vi "Dashboard Main.vi"() -> ()   [LabVIEW 2014]
uses:
  <vilib>/event_ctls.llb/eventvkey.ctl
  <vilib>/Rock Robotics/WPI/Dashboard/WPI_DashboardLogging Global.vi
  <vilib>/Utility/config.llb/Write Key (String).vi
  <vilib>/Utility/config.llb/Write Key (I32).vi
  <vilib>/Rock Robotics/Network Tables/SD Read Boolean.vi
  <vilib>/Rock Robotics/Network Tables/SD Write Number.vi
  <vilib>/Rock Robotics/Network Tables/SD Write Boolean.vi
  <vilib>/Utility/config.llb/NI_LVConfig.lvlib
panel:
  out "VISA resource name out":refnum<visa-resource-name>
  in  "TCP":refnum<k5>
  in  "Rec Mode":enum32{"Stop", "Record", "Playback"}(radio)
  in  "Vision":u16(ring) items=["Camera Off", "USB Camera SW", "USB Camera HW", "IP Camera"]
  out "Image Message":string="Timeout in Camera Communications"
  in  "Dashboard Tab":T1(tab)
  in  "Camera Settings":T2={"Frame Rate"=30, "Compression"=30, "Size"=1} {"Frame Rate" scale=1.0..30.0; "Size" items=["640x480", "320x240", "160x120"]}
  out "MotorChart R":cluster{"Numeric":dbl, "Numeric":dbl}(graph)
  out "MotorChart L":T3(graph)
  out "MotorSliders R":cluster{"MotorSlide1":dbl, "MotorSlide2":dbl} {"MotorSlide2" scale=-1.0..1.0 scale format="%#_2e"; "MotorSlide1" scale=-1.0..1.0 scale format="%#_2e"}
  out "MotorSliders L":T4 {"MotorSlide4 2" scale=0.0..14.0 scale format="%#_2e"; "MotorSlide2" scale=-1.0..1.0 scale format="%#_2e"; "MotorSlide1" scale=-1.0..1.0 scale format="%#_2e"}
  out "Gyro":dbl(knob) scale=0.0..360.0
  out "JS1 Z":dbl(slide) scale=-1.0..1.0 scale format="%#_2e"
  out "JS1 Graph":cluster{"X":dbl, "Y":dbl}[](graph)
  out "JS1 Buttons":T5
  out "JS2 Z":dbl(slide) scale=-1.0..1.0 scale format="%#_2e"
  out "JS2 Graph":cluster{"X":dbl, "Y":dbl}[](graph)
  out "JS2 Buttons":T5
  out "Mode":T6(ring)=enum."Auto Disabled"
  in  "DB Camera Config":bool
  out "fps":dbl format="%#.1g"
  out "Mbps":dbl format="%#.1g"
  out "Mbps 2":bool
  in  "dashButton5":bool
  out "Camera IP":string
  out "Boolean 2":bool
  in  "DB/String 9":string
  in  "DB/String 8":string
  in  "DB/String 7":string
  in  "DB/String 6":string
  in  "DB/String 5":string
  in  "DB/String 4":string
  in  "DB/String 3":string
  in  "DB/String 2":string
  in  "DB/String 1":string
  in  "DB/String 0":string
  in  "DB/Slider 0":dbl(slide) scale=0.0..5.0
  in  "DB/Slider 1":dbl(slide) scale=0.0..5.0
  in  "DB/Slider 2":dbl(slide) scale=0.0..5.0
  in  "DB/Slider 3":dbl(slide) scale=0.0..5.0
  out "DB/LED 3":bool
  out "DB/LED 2":bool
  out "DB/LED 1":bool
  out "DB/LED 0":bool
  in  "DB/Button 3":bool
  in  "DB/Button 2":bool
  in  "DB/Button 1":bool
  in  "DB/Button 0":bool caption="New Name"
  out "error out":errorcluster
  in  "Test Slider":dbl(slide) scale=0.0..100.0 scale format="%#_3g"
  in  "On/Off":bool caption="Solenoid"
  in  "Test Name":u16(ring) items=["Select the test to run...", "Example Test", "-------------------------------", "List of tests is built in robot code.", "Replace with your own automated tests."]
  in  "Test Tree":string(tree)
  in  "Motor":cluster{"Value":dbl, "Enable":bool} {"Value" scale=-1.0..1.0 scale format="%#_3g"}
  out "Progress":T7 {"Test Progress" scale=0.0..100.0}
  in  "Rev/Fwd":cluster{"Forward":bool, "Reverse":bool}
  in  "Test Ring":u16(ring) items=["Monochrome", "Color"]
  in  "Listbox":i32(listbox)
  out "Tree":string(tree)
  out "Camera Image":T8(plugin-control)
  out "Boolean":bool
  # "Left"
  # "Front"
  # "Right"
  # "Battery"
  # "test projectY"
  # "This tab is a great place for autonomous settings and robot-specific values.\nPlace controls and indicators inside this tab and match name to\nDashboard Variables on robot. You can also delete this comment."
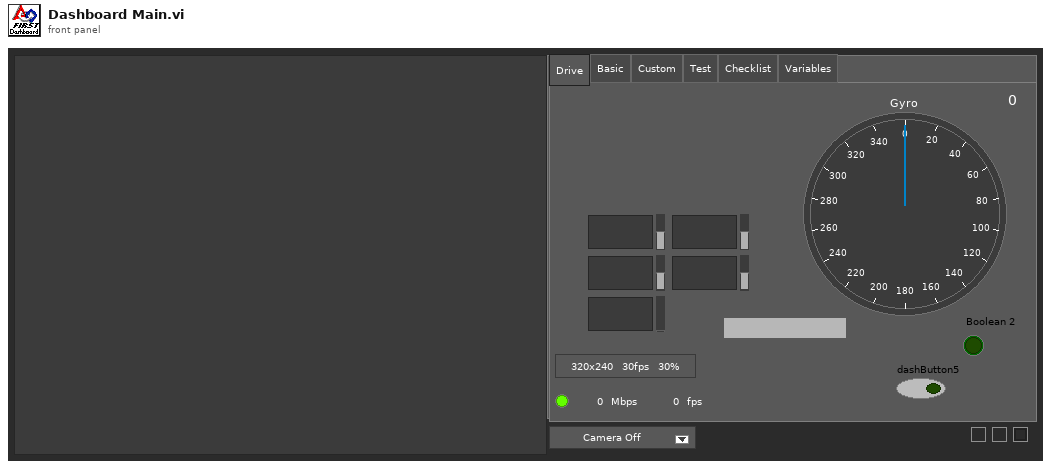
[diagram p1: front panel]
types:
  T1 = enum32{"Drive", "Basic", "Custom", "Test", "Checklist", "Variables"}
  T2 = cluster{"Frame Rate":i32, "Compression":i32, "Size":u16}
  T3 = cluster{"Numeric":dbl, "Numeric":dbl, "Battery V":dbl}
  T4 = cluster{"MotorSlide1":dbl, "MotorSlide2":dbl, "MotorSlide4 2":dbl}
  T5 = cluster{bool, bool, bool, bool, bool, bool, bool, bool, bool, bool, bool, bool}
  T6 = enum8{"Tele-Op Disabled", "Tele-Op Enabled", "Auto Disabled", "Auto Enabled", "Test Disabled", "Test Enabled", "Disconnected", "No Code", "E-Stop"}
  T7 = cluster{"Test Progress":u8, "Test Progress Text":string}
  T8 = typedef "IMAQ Image.ctl" = refnum<image>
  T9 = typedef "Image Type" = u32
  T10 = cluster{"Camera Image":refnum<vi>, "Dashboard Tab":refnum<vi>, "Boolean":refnum<vi>, "Vision":refnum<vi>, "Rec Mode":refnum<vi>, "Test Slider":refnum<vi>, "On/Off ":refnum<vi>, "Test Ring":refnum<vi>, "Rev/Fwd":refnum<vi>, "Test Name":refnum<vi>, "Motor":refnum<vi>, "Progress":refnum<vi>, "CheckList":refnum<vi>, "Tree":refnum<vi>, "Test Tree":refnum<vi>}
  T11 = cluster{"Error Strings":string, "Disable Counts":cluster{u16, u16}, "Rail Faults":cluster{u16, u16, u16}, "Robot IP":string, "DB Mode":u8, "Event Info":cluster{"Name":string, "Type":u8, "Number":u16, "Replay":u8}, "Camera Addr":string}
  T12 = cluster{"Storage":cluster{"Disk Free":u64, "RAM Block":u32, "RAM free":u32}, "CPU Utilization":cluster{"CPU % ISR":sgl, "CPU % Time Crit":sgl, "CPU % Timed Str":sgl, "CPU % High":sgl, "CPU % Above":sgl, "CPU % Normal":sgl, "CPU % Low":sgl}, "CAN":cluster{"% Bus Utilization":sgl, "Bus Off Cnt":u32, "TX_FIFO Full Cnt":u32, "Receive Error Cnt":u8, "Transmit Error Cnt":u8}, "HID":cluster{"HID Outputs":u32, "Rumble Low":u16, "Rumble High":u16}[]}
  T13 = cluster{"Status bits":cluster{"Test Mode":bool, "Autonomous":bool, "Enabled":bool, "Code Start":bool, "Brownout":bool, "Reserved 2":bool, "Reserved 3":bool, "E-Stop":bool}, "Code Trace":cluster{"Disabled":bool, "TeleOp":bool, "Auto":bool, "Test":bool}, "Controller Type":enum16{"unknown", "cRIO", "roboRio"}, "Code?":enum16{"unknown", "noCode", "code"}, "Battery V":dbl}
  T14 = cluster{"Control Bits":cluster{"TestMode":bool, "Autonomous":bool, "Enabled":bool, "FMS Present":bool, bool, bool, bool, "E-Stop":bool}, "Team Station ":u8, "Countdown":sgl, "Joystick Values":cluster{"Axes":dbl[], "Buttons":bool[], "POVs":i16[]}[]}
  T15 = cluster{"Axes":dbl[], "Buttons":bool[], "POVs":i16[]}[]
  T16 = cluster{"Axes":dbl[], "Buttons":bool[], "POVs":i16[]}
  T17 = cluster{"Buttons[0]":bool, "Buttons[1]":bool, "Buttons[2]":bool, "Buttons[3]":bool, "Buttons[4]":bool, "Buttons[5]":bool, "Buttons[6]":bool, "Buttons[7]":bool, "Buttons[8]":bool, "Buttons[9]":bool, "Buttons[10]":bool, "Buttons[11]":bool}
  T18 = cluster{"pickup":dbl, "1tote":dbl, "2tote":dbl, "3tote":dbl, "1container":dbl, "1container1tote":dbl, "1container2tote":dbl, "1container3tote":dbl}
  T19 = typedef "NI_LVConfig.lvlib/Config Data RefNum.ctl" = refnum<k1>
  T20 = cluster{"Operation":enum16{"Update", "Clear"}, "Color Box":u32}[]
  T21 = typedef "eventvkey.ctl" = enum16{"ASCII", "Enter", "Return", "Shift", "Ctrl", "Alt", "Cmd", "Opt", "Caps", "NumLock", "Clear", "Break", "Up", "Down", "Left", "Right", "Insert", "Delete", "Home", "End", "PageUp", "PageDown", "Escape", "Help", "Pause", "ScrollLock", "F1", "F2", "F3", "F4", "F5", "F6", "F7", "F8", "F9", "F10", "F11", "F12", "F13", "F14", "F15", "F16", "F17", "F18", "F19", "F20", "F21", "F22", "F23", "F24", "Play", "VolumeUp", "VolumeDown", "Mute", "Two Byte Char"}
  T22 = cluster{"Image Size":bool, "Image Type":bool, "Pixel Value":bool, "ROI Information":bool, "Zoom Factor":bool}
  T23 = enum8{"Enabled", "Disabled", "Disabled and Grayed Out"}
  T24 = cluster{"Operation":enum16{"Update", "Clear"}, "Color Box":u32}
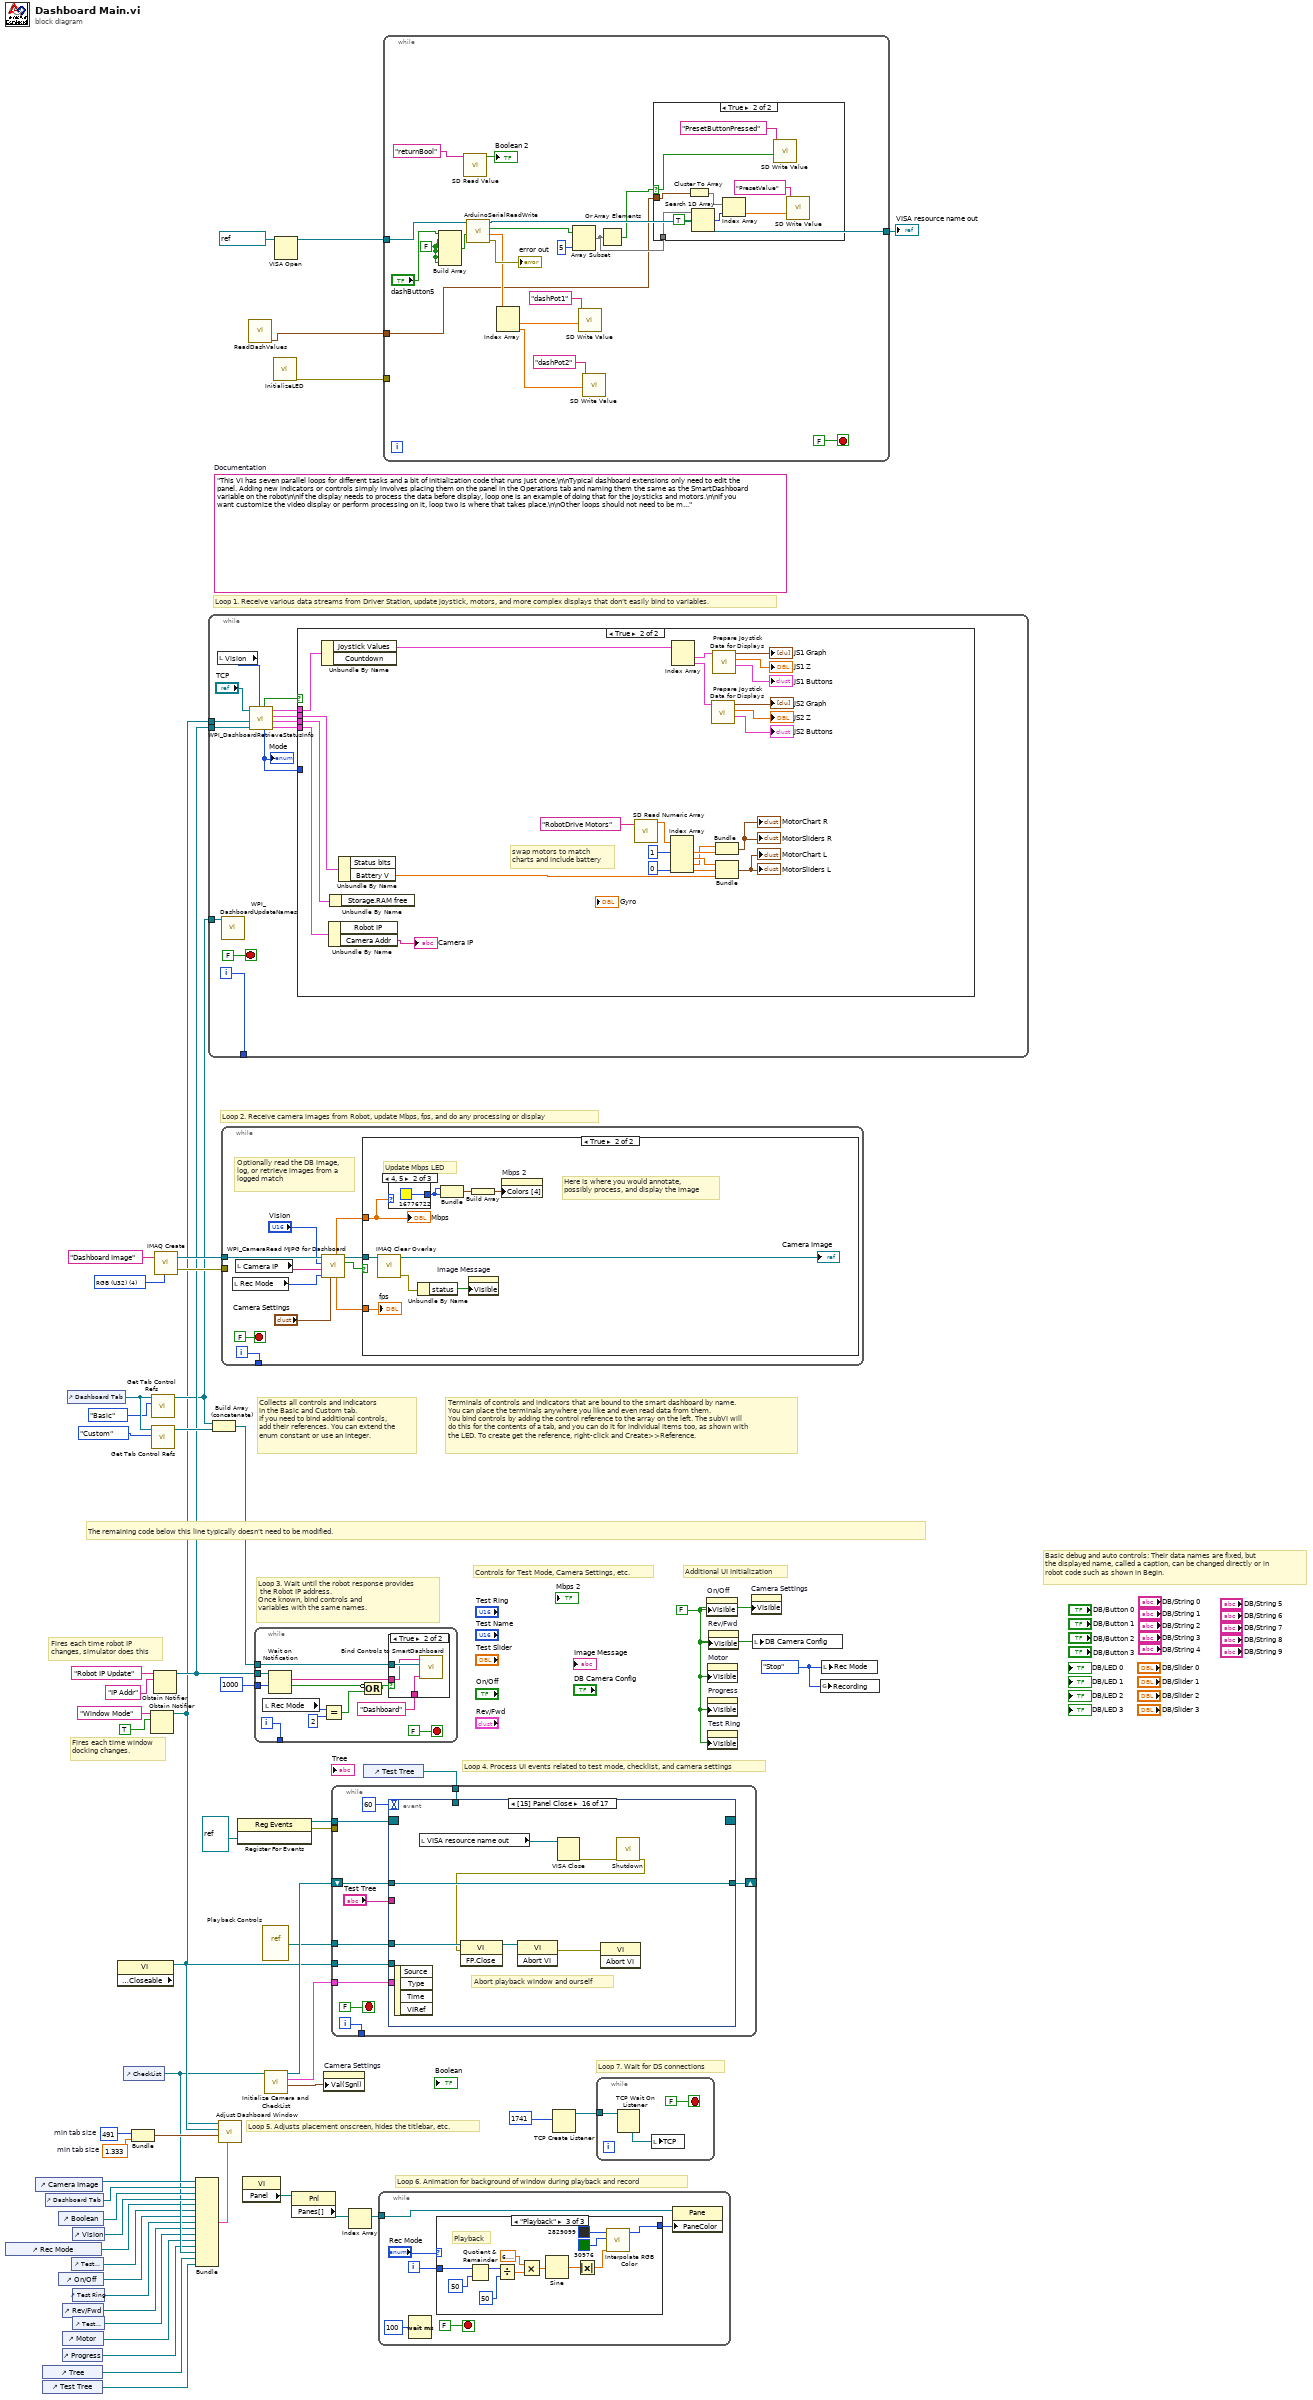
[diagram p0: block diagram]
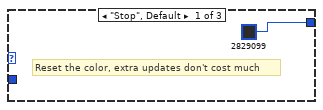
[diagram p4: hidden frame]
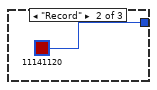
[diagram p5: hidden frame]
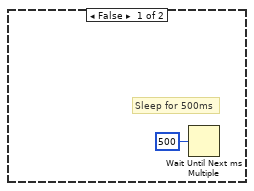
[diagram p7: hidden frame]
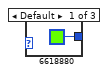
[diagram p8: hidden frame]
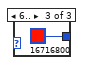
[diagram p9: hidden frame]
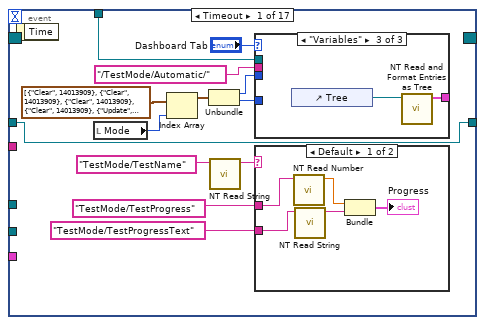
[diagram p10: hidden frame]
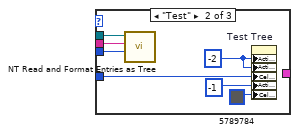
[diagram p12: hidden frame]
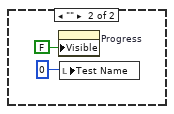
[diagram p13: hidden frame]
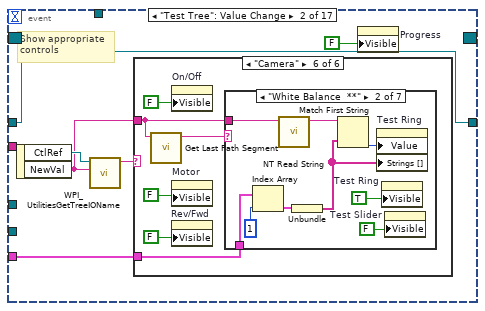
[diagram p14: hidden frame]
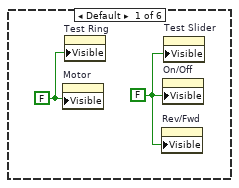
[diagram p15: hidden frame]
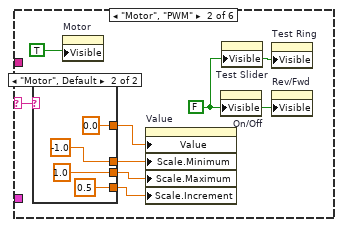
[diagram p16: hidden frame]
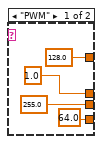
[diagram p17: hidden frame]
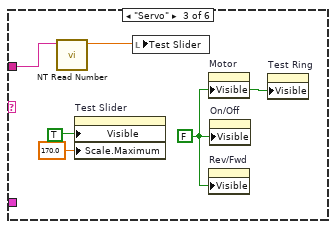
[diagram p18: hidden frame]
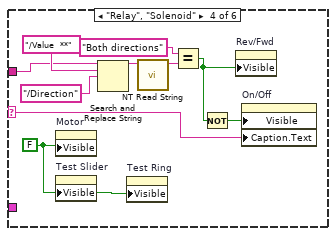
[diagram p19: hidden frame]
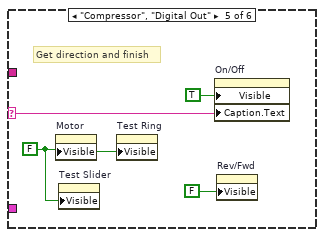
[diagram p20: hidden frame]
diagram:
  w29 = 491  # min tab size
  w28 = 1.333  # min tab size
  w37 = enum32{"Stop", "Record", "Playback"}."Stop" ("Rec Mode")
  w11 = FALSE ("Visible")
  (unwired) "This VI has seven parallel loops for different tasks and a bit of initialization code that runs just once.\n\nTypical dashboard extensions only need to edit the panel. Adding new indicators or controls simply involves placing them on the panel in the Operations tab and naming them the same as the SmartDashboard variable on the robot\n\nIf the display needs to process the data before display, loop one is an example of doing that for the joysticks and motors.\n\nIf you want customize the video display or perform processing on it, loop two is where that takes place.\n\nOther loops should not need to be modified. They are pretty standard, and document the task they perform."  # Documentation
  w57 = T9 4 items=["Grayscale (U8)", "Grayscale (I16)", "Grayscale (SGL)", "Complex (CSG)", "RGB (U32)", "HSL (U32)", "RGB (U64)"] ("Image Type")
  # "Loop 7. Wait for DS connections"
  # "Basic debug and auto controls: Their data names are fixed, but\nthe displayed name, called a caption, can be changed directly or in\nrobot code such as shown in Begin."
  # "Controls for Test Mode, Camera Settings, etc."
  # "Additional UI Initialization"
  # "Loop 6. Animation for background of window during playback and record"
  # "Fires each time robot IP\nchanges, simulator does this"
  # "Fires each time window\ndocking changes."
  # "Collects all controls and indicators\nin the Basic and Custom tab.\nIf you need to bind additional controls,\nadd their references. You can extend the\nenum constant or use an integer."
  # "The remaining code below this line typically doesn't need to be modified."
  # "Loop 4. Process UI events related to test mode, checklist, and camera settings"
  # "Terminals of controls and indicators that are bound to the smart dashboard by name.\nYou can place the terminals anywhere you like and even read data from them.\nYou bind controls by adding the control reference to the array on the left. The subVI will\ndo this for the contents of a tab, and you can do it for individual items too, as shown with\nthe LED. To create get the reference, right-click and Create>>Reference."
  # "Loop 3. Wait until the robot response provides\n the Robot IP address.\nOnce known, bind controls and\nvariables with the same names."
  # "Loop 5. Adjusts placement onscreen, hides the titlebar, etc."
  # "Loop 1. Receive various data streams from Driver Station, update joystick, motors, and more complex displays that don't easily bind to variables."
  # "Loop 2. Receive camera images from Robot, update Mbps, fps, and do any processing or display"
  n1 = control-ref of="Rec Mode"() -> (w17:refnum<vi>)
  n2 = control-ref of="Camera Image"() -> (w32:refnum<vi>)
  n3 = control-ref of="Tree"() -> (w21:refnum<vi>)
  n4 = control-ref of="Test Tree"() -> (w20:refnum<vi>)
  n5 = control-ref of="Dashboard Tab"() -> (w31:refnum<vi>)
  n6 = control-ref of="Boolean"() -> (w26:refnum<vi>)
  n7 = control-ref of="On/Off"() -> (w15:refnum<vi>)
  n8 = control-ref of="Progress"() -> (w12:refnum<vi>)
  n9 = control-ref of="Rev/Fwd"() -> (w13:refnum<vi>)
  n10 = control-ref of="Motor"() -> (w18:refnum<vi>)
  n11 = control-ref of="Dashboard Tab"() -> (w35:refnum<vi>)
  n12 = control-ref of="Test Slider"() -> (w16:refnum<vi>)
  n13 = control-ref of="Vision"() -> (w30:refnum<vi>)
  n14 = control-ref of="Test Ring"() -> (w14:refnum<vi>)
  n15 = control-ref of="Test Name"() -> (w19:refnum<vi>)
  n16 = property class="VI" props=["Front Panel.Closeable"]() -> (reference out=w36:refnum<vi>)  [unwired: 2 in, 2 out]
  n17 = control-ref of="CheckList"() -> (w22:refnum<vi>)
  n18 = Bundle("min tab size"=w29, "min tab size"=w28) -> (w27:cluster{"min tab size":i32, "min tab size":dbl})  [unwired: 1 in]
  n19 = Obtain Notifier(name (unnamed)="Window Mode", notification data type=TRUE) -> (notifier out=w8:refnum<notifier>)  [unwired: 2 in, 2 out]
  n20 = call <vilib>:"Get Tab Control Refs.vi"("Page Index"=T1."Basic" ("Dashboard Tab"), "TabControl in"=w35) -> ("ControlsOnPage"=w9:refnum<vi>[])  [unwired: 9 in]
  n21 = call <vilib>:"Get Tab Control Refs.vi"("Page Index"=T1."Custom" ("Dashboard Tab"), "TabControl in"=w35) -> ("ControlsOnPage"=w34:refnum<vi>[])  [unwired: 9 in]
  n22 = Obtain Notifier(name (unnamed)="Robot IP Update", notification data type="IP Addr" ("name (unnamed)")) -> (notifier out=w10:refnum<notifier>)  [unwired: 2 in, 2 out]
  n23 = call "IMAQ Create"("Image Name"="Dashboard Image", "Image Type"=w57) -> ("New Image"=w55:T8, "error out"=w54:errorcluster)  [unwired: 2 in, 1 out]
  n24 = Bundle("Camera Image"=w32, "Dashboard Tab"=w31, "Boolean"=w26, "Vision"=w30, "Rec Mode"=w17, "Test Slider"=w16, "On/Off"=w15, "Test Ring"=w14, "Rev/Fwd"=w13, "Test Name"=w19, "Motor"=w18, "Progress"=w12, "CheckList"=w22, "Tree"=w21, "Test Tree"=w20) -> (w23:T10)  [unwired: 1 in]
  n25 = while {
    tunnel: [w69] -> _
    tunnel: w10 -> [w63]
    tunnel: w9 -> [w62]
    tunnel: w8 -> [w58]
    i -> [w69]
    stop <- FALSE stop-if-true
    n26 = local read "Vision"() -> (w60:u16)
    n27 = call <vilib>:"WPI_DashboardUpdateNames.vi"("Controls on Tab"=w62) -> ()  [unwired: 11 in]
    n28 = call <vilib>:"WPI_DashboardRetrieveStatusInfo.vi"("Vision"=w60, "Binding Refnum"=w63, "Window Mode Notifier"=w58, "TCP Cnx"="TCP") -> ("Power and Errors"=w64:T11, "Robot Metrics"=w67:T12, "Status Info"=w68:T13, "Control Info"=w65:T14, "Robot Mode"=w61:T6, "Process?"=w66:bool)  [unwired: 2 in]
    "Mode" <- w61
    n29 = case shown="True" w66 {
      tunnel: w68 -> [_ w95]
      tunnel: w67 -> [_ w94]
      tunnel: w65 -> [_ w93]
      tunnel: w64 -> [_ w92]
      tunnel: w61 -> [_ _]
      frame False {
      }
      frame True {
        # "swap motors to match\ncharts and include battery"
        n30 = Unbundle By Name(w93) -> ("Joystick Values"=w80:T15)  [unwired: 1 out]
        n31 = Unbundle By Name(w92) -> ("Camera Addr"=→"Camera IP":string)  [unwired: 1 out]
        n32 = Unbundle By Name(w94) -> ()  [unwired: 1 out]
        n33 = Unbundle By Name(w95) -> ("Battery V"=w81:dbl)  [unwired: 1 out]
        n34 = call <vilib>:"SD Read Numeric Array.vi"("Name"="RobotDrive Motors") -> ("Numeric Array"=w83:dbl[])  [unwired: 8 in, 2 out]
        n35 = Index Array(array=w83, index #1=1, index #4=0) -> (element #1=w87:dbl, element #2=w88:dbl, element #3=w86:dbl, element #4=w91:dbl)  [unwired: 2 in]
        n36 = Index Array(array=w80) -> (element #1=w79:T16, element #2=w74:T16)  [unwired: 2 in]
        n37 = call "Prepare Joystick Data for Displays.vi"("Joystick Values"=w74) -> ("Buttons"=→"JS2 Buttons":T17, "Z Axis"=→"JS2 Z":dbl, "Cartesian Data"=→"JS2 Graph":cluster{"X axis":dbl, "X axis":dbl}[])  [unwired: 8 in]
        n38 = call "Prepare Joystick Data for Displays.vi"("Joystick Values"=w79) -> ("Buttons"=→"JS1 Buttons":T17, "Z Axis"=→"JS1 Z":dbl, "Cartesian Data"=→"JS1 Graph":cluster{"X axis":dbl, "X axis":dbl}[])  [unwired: 8 in]
        n39 = Bundle("Numeric"=w86, "Numeric"=w87) -> (→"MotorChart R" →"MotorSliders R":cluster{"Numeric":dbl, "Numeric":dbl})  [unwired: 1 in]
        n40 = Bundle("Numeric"=w88, "Numeric"=w91, "Battery V"=w81) -> (→"MotorChart L" →"MotorSliders L":T3)  [unwired: 1 in]
      }
    }
  }
  n41 = Build Array (concatenate)(w9, w34) -> (w33:refnum<vi>[])
  n42 = call "Adjust Dashboard Window.vi"("Sizing Refnums"=w23, "Size Constraints"=w27, "VI"=w36, "Notifier in"=w8) -> ()  [unwired: 8 in]
  n43 = while {
    tunnel: w55 -> [w104]
    tunnel: w54 -> [_]
    tunnel: [w105] -> _
    i -> [w105]
    stop <- FALSE stop-if-true
    # "Optionally read the DB image,\nlog, or retrieve images from a\nlogged match"
    n44 = local read "Rec Mode"() -> (w98:enum32{"Stop", "Record", "Playback"})
    n45 = local read "Camera IP"() -> (w96:string)
    n46 = call <vilib>:"WPI_CameraRead MJPG for Dashboard.vi"("Camera Settings"="Camera Settings", "Rec Mode"=w98, "Camera IP"=w96, "Camera Mode"="Vision", "Refnum in"=w104) -> ("Active"=w102:bool, "Refnum out"=w103:T8, "FPS"=w101:dbl, "Bandwidth (Mbps)"=w100:dbl)  [unwired: 3 in]
    n47 = case shown="True" w102 {
      tunnel: w103 -> [_ w111]
      tunnel: w100 -> [_ w110]
      tunnel: w101 -> [_ w108]
      frame False {
        # "Sleep for 500ms"
        n48 = Wait Until Next ms Multiple(millisecond multiple=u32 500) -> ()  [unwired: 1 out]
      }
      frame True {
        # "Here is where you would annotate,\npossibly process, and display the image"
        # "Update Mbps LED"
        n49 = call "IMAQ Clear Overlay"("Image"=w111) -> ("error out"=w115:errorcluster, "Image Out"=→"Camera Image":T8)  [unwired: 2 in, 7 out]
        n50 = case shown="4, 5" w110 {
          tunnel: [u32 6618880 ("Color Box") u32 16776722 ("Color Box") u32 16716800 ("Color Box")] -> w112
          frame Default {
          }
          frame 4, 5 {
          }
          frame 6.. {
          }
        }
        n51 = Unbundle By Name(w115) -> ("status"=w116:bool)
        n52 = Bundle("Color Box"=w112, "Color Box"=w112) -> (w114:cluster{"Color Box":u32, "Color Box":u32})  [unwired: 1 out]
        n53 = property on="Image Message" class="Str"("Visible"=w116) -> ()  [unwired: 2 in, 2 out]
        n54 = Build Array(w114) -> (w113:cluster{"Color Box":u32, "Color Box":u32}[])
        n55 = property on="Mbps 2" class="Bool (strict)"("Colors [4]"=w113) -> ()  [unwired: 2 in, 2 out]
        "Mbps" <- w110
        "fps" <- w108
      }
    }
  }
  n56 = register-events(refnum<vi> refnum) -> (reference out=w41:refnum<event-registration>, error out=w40:errorcluster)  [unwired: 2 in]
  n57 = property class="VI"() -> ("Panel"=w44:refnum<vi>)  [unwired: 2 in, 2 out]
  n58 = call "ReadDashValues.vi"() -> ("output cluster"=w2:T18)  [unwired: 11 in]
  n59 = while {
    tunnel: w33 -> [w131]
    tunnel: w10 -> [w129]
    tunnel: [w127] -> _
    tunnel: u32 1000 ("milliseconds to wait") -> [w126]
    i -> [w127]
    stop <- FALSE stop-if-true
    n60 = local read "Rec Mode"() -> (w122:enum32{"Stop", "Record", "Playback"})
    n61 = Wait on Notification(notifier=w129, timeout in ms (-1)=w126) -> (notification=w128:string, timed out?=w124:bool)  [unwired: 2 in, 2 out]
    n62 = Equal?(x=w122, y=u16 2 ("Rec Mode")) -> (x = y?=w123:bool)
    n63 = Compound Arithmetic op=OR(invert w124, w123) -> (w125:bool)
    n64 = case shown="True" w125 {
      tunnel: w131 -> [_ w134]
      tunnel: w128 -> [_ w133]
      tunnel: "Dashboard" -> [_ w132]
      frame False {
      }
      frame True {
        n65 = call <vilib>:"Bind Controls to SmartDashboard.vi"("Client Name"=w132, "Bound Control Refs"=w134, "Server IP Address"=w133) -> ()  [unwired: 9 in]
      }
    }
  }
  n66 = vi-ref "Playback Controls.vi"() -> (w42:refnum<vi>)
  n67 = call "Initialize Camera and CheckList.vi"("ListBox in"=w22) -> ("Cluster"=w48:cluster{"value":i32, "value":i32, "index":i32}, "Array"=w49:cluster{string[]}[], "File Refnum"=w47:T19)  [unwired: 8 in]
  n68 = call "InitializeLED.vi"() -> ("error out"=w1:errorcluster)  [unwired: 11 in]
  n69 = VISA Open(VISA resource name=refnum<visa-resource-name> "COM3") -> (VISA resource name=w4:refnum<visa-resource-name>)  [unwired: 4 in, 1 out]
  n70 = property class="Pnl"(reference=w44) -> ("Panes[]"=w45:refnum<vi>[])  [unwired: 1 in, 2 out]
  n71 = property on="Camera Settings" class="Clust (strict)"("Val(Sgnl)"=w48) -> ()  [unwired: 2 in, 2 out]
  n72 = Index Array(array=w45) -> (element=w43:refnum<vi>)  [unwired: 1 in]
  n73 = control-ref of="Test Tree"() -> (w46:refnum<vi>)
  n74 = while {
    tunnel: w49 -> [w142]
    shift-right: [w141] -> _
    shift-left: w47 -> [w140]
    tunnel: [w139] -> _
    tunnel: w46 -> [w138]
    tunnel: w42 -> [w137]
    tunnel: w41 -> [w136]
    tunnel: w40 -> [_]
    tunnel: w36 -> [w135]
    i -> [w139]
    stop <- FALSE stop-if-true
    n75 = event shown="[15] Panel Close" {
      selector: w136 -> [_ _ _ _ _ _ _ _ _ _ _ _ _ _ _ _ _]
      dyn-events: [_ _ _ _ _ _ _ _ _ _ _ _ _ w380 _ _ _] -> _
      timeout: u32 60 ("milliseconds to wait") -> [_ _ _ _ _ _ _ _ _ _ _ _ _ _ _ _ _]
      tunnel: w138 -> [w154 _ _ _ _ _ _ _ _ _ _ _ _ _ _ _ _]
      tunnel: "Test Tree" -> [_ _ _ _ _ _ _ _ w349 w357 w359 w363 w371 _ _ _ _]
      tunnel: w142 -> [_ w176 _ _ _ _ w313 w343 _ _ _ _ _ _ _ _ _]
      tunnel: [w150 w175 w274 w279 w287 w299 w312 w336 w348 w355 w358 w362 w370 w382 w396 w400 w410] -> w141
      tunnel: w140 -> [w150 w175 w274 w279 w287 w299 w311 w336 w348 w355 w358 w362 w370 w382 w396 w400 w410]
      tunnel: w137 -> [_ _ _ _ _ _ _ _ _ _ _ _ _ w383 _ w403 _]
      tunnel: w135 -> [_ _ _ _ _ _ _ _ _ _ _ _ _ w378 _ _ _]
      event Timeout {
        n76 = event-data() -> ()  [unwired: 1 in, 1 out]
        n77 = local read "Mode"() -> (w153:T6)
        n78 = Index Array(array=T20 [{"Operation"=enum."Clear", "Color Box"=14013909}, {"Operation"=enum."Clear", "Color Box"=14013909}, {"Operation"=enum."Clear", "Color Box"=14013909}, {"Operation"=enum."Clear", "Color Box"=14013909}, {"Operation"=enum."Update", "Color Box"=14013909}, {"Operation"=enum."Update", "Color Box"=16777215}, {"Operation"=enum."Clear", "Color Box"=14013909}, {"Operation"=enum."Clear", "Color Box"=14013909}, {"Operation"=enum."Clear", "Color Box"=14013909}], index=w153) -> (element=w148:T24)
        n79 = Unbundle(w148) -> ("Operation"=w147:enum16{"Update", "Clear"}, "Color Box"=w146:u32)
        n80 = call <vilib>:"NT Read String.vi"("Name"="TestMode/TestName") -> ("String"=w157:string)  [unwired: 9 in, 1 out]
        n81 = case shown="\"Variables\"" "Dashboard Tab" {
          tunnel: w154 -> [_ w165 _]
          tunnel: "/TestMode/Automatic/" ("Name Pattern") -> [_ w164 _]
          tunnel: w147 -> [_ w163 _]
          tunnel: [_ _ w167] -> _
          tunnel: w146 -> [_ w159 _]
          frame "Custom", Default {
          }
          frame "Test" {
            w162 = -2 ("Active Item:Row Number")
            n82 = call <vilib>:"NT Read and Format Entries as Tree.vi"("Operation"=w163, "Name Pattern"=w164, "Tree Refnum"=w165) -> ()  [unwired: 7 in, 2 out]
            n83 = property on="Test Tree" class="Tree (strict)"("Active Item Row Number"=w162, "ActiveColNum"=w162, "CellBG"=w159, "Active Item Row Number"=-1 ("Active Item:Row Number"), "CellBG"=u32 5789784 ("Color Box")) -> ()  [unwired: 2 in, 2 out]
          }
          frame "Variables" {
            n84 = control-ref of="Tree"() -> (w166:refnum<vi>)
            n85 = call <vilib>:"NT Read and Format Entries as Tree.vi"("Tree Refnum"=w166) -> ("Formatted Strings"=w167:cluster{"Name":string, "Value":string}[])  [unwired: 9 in, 1 out]
          }
        }
        n86 = case shown="Default" w157 {
          tunnel: "TestMode/TestProgress" ("Name") -> [w169 _]
          tunnel: "TestMode/TestProgressText" ("Name") -> [w168 _]
          frame Default {
            n87 = call <vilib>:"NT Read Number.vi"("Name"=w169) -> ("Numeric"=w170:dbl)  [unwired: 9 in, 1 out]
            n88 = call <vilib>:"NT Read String.vi"("Name"=w168) -> ("String"=w171:string)  [unwired: 9 in, 1 out]
            n89 = Bundle("Numeric"=w170, "String"=w171) -> (→"Progress":cluster{"Numeric":dbl, "String":string})  [unwired: 1 in]
          }
          frame "" {
            n90 = property on="Progress" class="Clust (strict)"("Visible"=FALSE) -> ()  [unwired: 2 in, 2 out]
            n91 = local write "Test Name"(u16 0) -> ()
          }
        }
      }
      event "Test Tree": Value Change {
        # "Show appropriate\ncontrols"
        n92 = event-data() -> ("CtlRef"=w179:refnum<vi>, "NewVal"=w177:string)  [unwired: 1 in]
        n93 = call <vilib>:"WPI_UtilitiesGetTreeIOName.vi"("NewVal"=w177, "TreeControl in"=w179) -> ("I/O Name"=w180:string)  [unwired: 9 in]
        n94 = case shown="\"Camera\"" w180 {
          selector: w180 -> [_ w187 _ w205 w214 _]
          tunnel: w177 -> [_ _ w202 w204 _ w221]
          tunnel: w176 -> [_ _ _ _ _ w220]
          frame Default {
            w182 = FALSE ("Visible")
            w181 = FALSE ("Visible")
            n95 = property on="Motor" class="Clust (strict)"("Visible"=w181) -> ()  [unwired: 2 in, 2 out]
            n96 = property on="Test Ring" class="Ring (strict)"("Visible"=w181) -> ()  [unwired: 2 in, 2 out]
            n97 = property on="Rev/Fwd" class="Clust (strict)"("Visible"=w182) -> ()  [unwired: 2 in, 2 out]
            n98 = property on="On/Off" class="Bool (strict)"("Visible"=w182) -> ()  [unwired: 2 in, 2 out]
            n99 = property on="Test Slider" class="Slide (strict)"("Visible"=w182) -> ()  [unwired: 2 in, 2 out]
          }
          frame "Motor", "PWM" {
            w188 = FALSE ("Visible")
            n100 = case shown="\"Motor\", Default" w187 {
              tunnel: [1.0 ("Value") -1.0 ("Value")] -> w186
              tunnel: [255.0 ("Value") 1.0 ("Value")] -> w185
              tunnel: [128.0 ("Value") 0.0 ("Value")] -> w184
              tunnel: [64.0 ("Value") 0.5 ("Value")] -> w183
              frame "PWM" {
              }
              frame "Motor", Default {
              }
            }
            n101 = property on="Motor" class="Clust (strict)"("Visible"=TRUE) -> ()  [unwired: 2 in, 2 out]
            n102 = property on="Value" class="Slide (strict)"("Value"=w184, "Scale.Minimum"=w186, "Scale.Maximum"=w185, "Scale.Increment"=w183) -> ()  [unwired: 2 in, 2 out]
            n103 = property on="On/Off" class="Bool (strict)"("Visible"=w188) -> ()  [unwired: 2 in, 2 out]
            n104 = property on="Test Slider" class="Slide (strict)"("Visible"=w188) -> ()  [unwired: 2 in, 2 out]
            n105 = property on="Test Ring" class="Ring (strict)"("Visible"=w188) -> ()  [unwired: 2 in, 2 out]
            n106 = property on="Rev/Fwd" class="Clust (strict)"("Visible"=w188) -> ()  [unwired: 2 in, 2 out]
          }
          frame "Servo" {
            w200 = FALSE ("Visible")
            n107 = call <vilib>:"NT Read Number.vi"("Name"=w202) -> ("Numeric"=w201:dbl)  [unwired: 9 in, 1 out]
            n108 = property on="Test Slider" class="Slide (strict)"("Visible"=TRUE, "Scale.Maximum"=170.0 ("Scale.Range:Maximum")) -> ()  [unwired: 2 in, 2 out]
            n109 = local write "Test Slider"(w201) -> ()
            n110 = property on="Motor" class="Clust (strict)"("Visible"=w200) -> ()  [unwired: 2 in, 2 out]
            n111 = property on="Rev/Fwd" class="Clust (strict)"("Visible"=w200) -> ()  [unwired: 2 in, 2 out]
            n112 = property on="On/Off" class="Bool (strict)"("Visible"=w200) -> ()  [unwired: 2 in, 2 out]
            n113 = property on="Test Ring" class="Ring (strict)"("Visible"=w200) -> ()  [unwired: 2 in, 2 out]
          }
          frame "Relay", "Solenoid" {
            w203 = FALSE ("Visible")
            n114 = property on="Motor" class="Clust (strict)"("Visible"=w203) -> ()  [unwired: 2 in, 2 out]
            n115 = property on="Test Slider" class="Slide (strict)"("Visible"=w203) -> ()  [unwired: 2 in, 2 out]
            n116 = Search and Replace String(input string=w204, search string="/Value  **", replace string="/Direction") -> (result string=w210:string)  [unwired: 5 in, 3 out]
            n117 = property on="Test Ring" class="Ring (strict)"("Visible"=w203) -> ()  [unwired: 2 in, 2 out]
            n118 = call <vilib>:"NT Read String.vi"("Name"=w210) -> ("String"=w208:string)  [unwired: 9 in, 1 out]
            n119 = Equal?(x="Both directions", y=w208) -> (x = y?=w206:bool)
            n120 = Not(x=w206) -> (.not. x?=w207:bool)
            n121 = property on="Rev/Fwd" class="Clust (strict)"("Visible"=w206) -> ()  [unwired: 2 in, 2 out]
            n122 = property on="On/Off" class="Bool (strict)"("Visible"=w207, "Caption.Text"=w205) -> ()  [unwired: 2 in, 2 out]
          }
          frame "Compressor", "Digital Out" {
            w213 = FALSE ("Visible")
            # "Get direction and finish"
            n123 = property on="Motor" class="Clust (strict)"("Visible"=w213) -> ()  [unwired: 2 in, 2 out]
            n124 = property on="Test Slider" class="Slide (strict)"("Visible"=w213) -> ()  [unwired: 2 in, 2 out]
            n125 = property on="Test Ring" class="Ring (strict)"("Visible"=w213) -> ()  [unwired: 2 in, 2 out]
            n126 = property on="On/Off" class="Bool (strict)"("Visible"=TRUE, "Caption.Text"=w214) -> ()  [unwired: 2 in, 2 out]
            n127 = property on="Rev/Fwd" class="Clust (strict)"("Visible"=FALSE) -> ()  [unwired: 2 in, 2 out]
          }
          frame "Camera" {
            n128 = call <vilib>:"Get Last Path Segment.vi"("String in"=w221) -> ("String out"=w222:string)  [unwired: 10 in]
            n129 = property on="On/Off" class="Bool (strict)"("Visible"=FALSE) -> ()  [unwired: 2 in, 2 out]
            n130 = property on="Motor" class="Clust (strict)"("Visible"=FALSE) -> ()  [unwired: 2 in, 2 out]
            n131 = property on="Rev/Fwd" class="Clust (strict)"("Visible"=FALSE) -> ()  [unwired: 2 in, 2 out]
            n132 = case shown="\"White Balance  **\"" w222 {
              tunnel: w221 -> [w228 w237 w246 w255 w264 _ w270]
              tunnel: w220 -> [w226 w234 w243 w252 w261 _ _]
              frame "Size  **" {
                n133 = Index Array(array=w226) -> (element=w225:cluster{string[]})  [unwired: 1 in]
                n134 = call <vilib>:"NT Read String.vi"("Name"=w228) -> ("String"=w227:string)  [unwired: 9 in, 1 out]
                n135 = Unbundle(w225) -> (w223:string[])
                n136 = Match First String(2:w223, 3:w227) -> (0:w224:i32)  [unwired: 1 out]
                n137 = property on="Test Ring" class="Ring (strict)"("Value"=w224, "Strings []"=w223) -> ()  [unwired: 2 in, 2 out]
                n138 = property on="Test Ring" class="Ring (strict)"("Visible"=TRUE) -> ()  [unwired: 2 in, 2 out]
                n139 = property on="Test Slider" class="Slide (strict)"("Visible"=FALSE) -> ()  [unwired: 2 in, 2 out]
              }
              frame "White Balance  **" {
                n140 = Index Array(array=w234, index=1) -> (element=w235:cluster{string[]})
                n141 = call <vilib>:"NT Read String.vi"("Name"=w237) -> ("String"=w236:string)  [unwired: 9 in, 1 out]
                n142 = Unbundle(w235) -> (w232:string[])
                n143 = Match First String(2:w232, 3:w236) -> (0:w231:i32)  [unwired: 1 out]
                n144 = property on="Test Ring" class="Ring (strict)"("Value"=w231, "Strings []"=w232) -> ()  [unwired: 2 in, 2 out]
                n145 = property on="Test Ring" class="Ring (strict)"("Visible"=TRUE) -> ()  [unwired: 2 in, 2 out]
                n146 = property on="Test Slider" class="Slide (strict)"("Visible"=FALSE) -> ()  [unwired: 2 in, 2 out]
              }
              frame "Exposure  **" {
                n147 = Index Array(array=w243, index=2) -> (element=w244:cluster{string[]})
                n148 = call <vilib>:"NT Read String.vi"("Name"=w246) -> ("String"=w245:string)  [unwired: 9 in, 1 out]
                n149 = Unbundle(w244) -> (w240:string[])
                n150 = Match First String(2:w240, 3:w245) -> (0:w241:i32)  [unwired: 1 out]
                n151 = property on="Test Ring" class="Ring (strict)"("Value"=w241, "Strings []"=w240) -> ()  [unwired: 2 in, 2 out]
                n152 = property on="Test Ring" class="Ring (strict)"("Visible"=TRUE) -> ()  [unwired: 2 in, 2 out]
                n153 = property on="Test Slider" class="Slide (strict)"("Visible"=FALSE) -> ()  [unwired: 2 in, 2 out]
              }
              frame "Exposure Priority  **" {
                n154 = Index Array(array=w252, index=3) -> (element=w253:cluster{string[]})
                n155 = call <vilib>:"NT Read String.vi"("Name"=w255) -> ("String"=w254:string)  [unwired: 9 in, 1 out]
                n156 = Unbundle(w253) -> (w249:string[])
                n157 = Match First String(2:w249, 3:w254) -> (0:w250:i32)  [unwired: 1 out]
                n158 = property on="Test Ring" class="Ring (strict)"("Value"=w250, "Strings []"=w249) -> ()  [unwired: 2 in, 2 out]
                n159 = property on="Test Ring" class="Ring (strict)"("Visible"=TRUE) -> ()  [unwired: 2 in, 2 out]
                n160 = property on="Test Slider" class="Slide (strict)"("Visible"=FALSE) -> ()  [unwired: 2 in, 2 out]
              }
              frame "Color Enable  **" {
                n161 = Index Array(array=w261, index=4) -> (element=w262:cluster{string[]})
                n162 = call <vilib>:"NT Read String.vi"("Name"=w264) -> ("String"=w263:string)  [unwired: 9 in, 1 out]
                n163 = Unbundle(w262) -> (w258:string[])
                n164 = Match First String(2:w258, 3:w263) -> (0:w259:i32)  [unwired: 1 out]
                n165 = property on="Test Ring" class="Ring (strict)"("Value"=w259, "Strings []"=w258) -> ()  [unwired: 2 in, 2 out]
                n166 = property on="Test Ring" class="Ring (strict)"("Visible"=TRUE) -> ()  [unwired: 2 in, 2 out]
                n167 = property on="Test Slider" class="Slide (strict)"("Visible"=FALSE) -> ()  [unwired: 2 in, 2 out]
              }
              frame Default {
                n168 = property on="Test Ring" class="Ring (strict)"("Visible"=FALSE) -> ()  [unwired: 2 in, 2 out]
                n169 = property on="Test Slider" class="Slide (strict)"("Visible"=FALSE) -> ()  [unwired: 2 in, 2 out]
              }
              frame "Brightness  **", "Color Level  **", "Compression  **", "FPS  **", "Sharpness  **" {
                n170 = call <vilib>:"NT Read Number.vi"("Name"=w270) -> ("Numeric"=w269:dbl)  [unwired: 9 in, 1 out]
                n171 = local write "Test Slider"(w269) -> ()
                n172 = property on="Test Slider" class="Slide (strict)"("Visible"=TRUE, "Scale.Maximum"=100.0 ("Scale.Range:Maximum")) -> ()  [unwired: 2 in, 2 out]
                n173 = property on="Test Ring" class="Ring (strict)"("Visible"=FALSE) -> ()  [unwired: 2 in, 2 out]
              }
            }
          }
        }
        n174 = property on="Progress" class="Clust (strict)"("Visible"=FALSE) -> ()  [unwired: 2 in, 2 out]
      }
      event "Test Name": Mouse Enter {
        # "Populate the ring with the list of tests"
        n175 = event-data() -> ()  [unwired: 1 in, 1 out]
        n176 = call <vilib>:"NT Read String Array.vi"("Name"="TestMode/TestList") -> ("String Array"=w278:string[])  [unwired: 9 in, 1 out]
        n177 = Build Array (concatenate)("Select the test to run...", w278) -> (w277:string[])
        n178 = property on="Test Name" class="Ring (strict)"("Strings []"=w277) -> ()  [unwired: 2 in, 2 out]
      }
      event "Test Name": Value Change {
        w280 = FALSE ("Visible")
        # "Tell the robot the test name to run"
        n179 = event-data() -> ("NewVal"=w284:u16)  [unwired: 1 in]
        n180 = property on="Test Name" class="Ring (strict)"() -> ("Strings []"=w285:string[])  [unwired: 2 in, 2 out]
        n181 = local write "Progress"(T7 {"Test Progress"=0, "Test Progress Text"=""} ("Progress")) -> ()
        n182 = Index Array(array=w285, index=w284) -> (element=w283:string)
        n183 = call <vilib>:"NT Write String.vi"("String"=w283, "Name"="TestMode/TestName") -> ()  [unwired: 9 in, 1 out]
        n184 = property on="Progress" class="Clust (strict)"("Visible"=TRUE) -> ()  [unwired: 2 in, 2 out]
        n185 = property on="Motor" class="Clust (strict)"("Visible"=w280) -> ()  [unwired: 2 in, 2 out]
        n186 = property on="Test Slider" class="Slide (strict)"("Visible"=w280) -> ()  [unwired: 2 in, 2 out]
        n187 = property on="On/Off" class="Bool (strict)"("Visible"=w280) -> ()  [unwired: 2 in, 2 out]
        n188 = property on="Rev/Fwd" class="Clust (strict)"("Visible"=w280) -> ()  [unwired: 2 in, 2 out]
        n189 = property on="Test Ring" class="Ring (strict)"("Visible"=w280) -> ()  [unwired: 2 in, 2 out]
      }
      event "Listbox": Double Click {
        # "Shift clears all"
        # "Update symbols on the listbox"
        n190 = event-data() -> ("PlatMods.Shift"=w288:bool, "Row"=w290:i32)  [unwired: 1 in]
        n191 = case shown="True" w288 {
          tunnel: w290 -> [w294 _]
          tunnel: 1 -> [w293 _]
          frame False {
            n192 = property on="Listbox" class="LstBox (strict)"() -> ("Item Symbols"=w292:i32[])  [unwired: 2 in, 2 out]
            n193 = Replace Array Subset(array=w292, new element=w293, index=w294) -> (w291:i32[])
            n194 = property on="Listbox" class="LstBox (strict)"("Item Symbols"=w291) -> ()  [unwired: 2 in, 2 out]
          }
          frame True {
            w295 = 0 ("Top Row")
            n195 = property on="Listbox" class="LstBox (strict)"() -> ("Number of Rows"=w297:u32)  [unwired: 2 in, 2 out]
            n196 = Initialize Array(0, w297) -> (w296:i32[])
            n197 = property on="Listbox" class="LstBox (strict)"("Top Row"=w295, "Value"=w295, "Item Symbols"=w296) -> ()  [unwired: 2 in, 2 out]
          }
        }
      }
      event "Listbox": Key Down {
        # "Update symbols on the listbox\nLeft and right keys check and uncheck"
        n198 = event-data() -> ("VKey"=w301:T21)  [unwired: 1 in]
        n199 = case shown="\"Left\", \"Right\"" w301 {
          selector: w301 -> [w306 _]
          tunnel: eventvkey."Left" ("VKey") -> [w304 _]
          frame "Left", "Right" {
            n200 = Equal?(x=w304, y=w306) -> (x = y?=w305:bool)
            n201 = Select(t=0, s=w305, f=1) -> (s? t:f=w307:i32)
            n202 = property on="Listbox" class="LstBox (strict)"() -> ("Item Symbols"=w310:i32[])  [unwired: 2 in, 2 out]
            n203 = Replace Array Subset(array=w310, new element=w307, index="Listbox") -> (w309:i32[])
            n204 = property on="Listbox" class="LstBox (strict)"("Item Symbols"=w309) -> ()  [unwired: 2 in, 2 out]
          }
          frame Default {
          }
        }
      }
      event "DB Camera Config": Value Change {
        # "Show or hide the cluster of controls, store in ini file"
        n205 = event-data() -> ("NewVal"=w314:bool)  [unwired: 1 in]
        n206 = case shown="False" w314 {
          tunnel: w313 -> [w323 _]
          tunnel: [w316 w334] -> w312
          tunnel: w311 -> [w315 w334]
          frame False {
            w330 = "Camera"
            w333 = FALSE ("Visible")
            n207 = local read "Camera Settings"() -> (w322:T2)
            n208 = Index Array(array=w323) -> (element=w326:cluster{string[]})  [unwired: 1 in]
            n209 = Unbundle(w322) -> ("Frame Rate"=w321:i32, "Compression"=w320:i32, "Size"=w324:u16)
            n210 = Unbundle(w326) -> (w325:string[])
            n211 = Index Array(array=w325, index=w324) -> (element=w319:string)
            n212 = call-poly <vilib>:"Write Key.vi"("section"=w330, "value"=w319, "key"="Size", "refnum"=w315) -> ("refnum out"=w332:T19)  [unwired: 2 in, 5 out]
            n213 = call-poly <vilib>:"Write Key.vi"("section"=w330, "value"=w321, "key"="FrameRate", "refnum"=w332) -> ("refnum out"=w331:T19)  [unwired: 1 in, 6 out]
            n214 = property on="Camera Settings" class="Clust (strict)"("Visible"=w333) -> ()  [unwired: 2 in, 2 out]
            n215 = local write "DB Camera Config"(w333) -> ()
            n216 = call-poly <vilib>:"Write Key.vi"("section"=w330, "value"=w320, "key"="Compression", "refnum"=w331) -> ("refnum out"=w317:T19)  [unwired: 1 in, 6 out]
            n217 = call <vilib>:"Close Config Data.vi"("refnum"=w317) -> ("file path"=w318:path)  [unwired: 2 in, 8 out]
            n218 = call <vilib>:"Open Config Data.vi"("configuration file path"=w318) -> ("refnum"=w316:T19)  [unwired: 8 in, 2 out]
          }
          frame True {
            n219 = property on="Camera Settings" class="Clust (strict)"("Visible"=TRUE) -> ()  [unwired: 2 in, 2 out]
          }
        }
      }
      event "Camera Settings": Value Change {
        # "Update summary string when any elements of DB camera change"
        n220 = event-data() -> ("NewVal"=w347:T2)  [unwired: 1 in]
        n221 = Index Array(array=w343) -> (element=w342:cluster{string[]})  [unwired: 1 in]
        n222 = Unbundle(w347) -> ("Frame Rate"=w338:i32, "Compression"=w337:i32, "Size"=w340:u16)
        n223 = Unbundle(w342) -> (w341:string[])
        n224 = Index Array(array=w341, index=w340) -> (element=w339:string)
        n225 = Format Into String(format string="%s   %dfps   %d%%", w339, w338, w337) -> (resulting string=w344:string)  [unwired: 2 in, 1 out]
        n226 = Build Array(w344) -> (w345:string[])
        n227 = property on="DB Camera Config" class="Bool (strict)"("Strings [4]"=w345) -> ()  [unwired: 2 in, 2 out]
      }
      event "Motor.Enable": Value Change {
        # "When the test mode otor enable helper is set, update that\ntree row item's value"
        n228 = event-data() -> ("NewVal"=w353:bool)  [unwired: 1 in]
        n229 = Unbundle("Motor") -> ("Value"=w352:dbl)  [unwired: 1 out]
        n230 = Select(t=w352, s=w353, f=0.0) -> (s? t:f=w350:dbl)
        n231 = call <vilib>:"NT Write Number.vi"("Numeric"=w350, "Name"=w349) -> ()  [unwired: 9 in, 1 out]
      }
      event "Test Slider": Value Change {
        # "When the test mode slider helper is set, update that\ntree row item's value"
        n232 = event-data() -> ("NewVal"=w356:dbl)  [unwired: 1 in]
        n233 = call <vilib>:"NT Write Number.vi"("Numeric"=w356, "Name"=w357) -> ()  [unwired: 9 in, 1 out]
      }
      event "On/Off": Value Change {
        # "When the test mode on/off helper value is set, update that\ntree row item's value"
        n234 = event-data() -> ("NewVal"=w361:bool)  [unwired: 1 in]
        n235 = Boolean To (0,1)(Boolean=w361) -> (0, 1=w360:i16)
        n236 = call <vilib>:"NT Write Number.vi"("Numeric"=w360, "Name"=w359) -> ()  [unwired: 9 in, 1 out]
      }
      event "Rev/Fwd": Value Change {
        # "When the test mode helper value for relays is set, update that\ntree row item's value"
        n237 = event-data() -> ("NewVal.Forward"=w369:bool, "NewVal.Reverse"=w368:bool)  [unwired: 1 in]
        n238 = Boolean To (0,1)(Boolean=w369) -> (0, 1=w365:i16)
        n239 = Boolean To (0,1)(Boolean=w368) -> (0, 1=w367:i16)
        n240 = Negate(x=w367) -> (-x=w366:i16)
        n241 = Add(x=w365, y=w366) -> (x+y=w364:i16)
        n242 = call <vilib>:"NT Write Number.vi"("Numeric"=w364, "Name"=w363) -> ()  [unwired: 9 in, 1 out]
      }
      event "Test Ring": Value Change {
        # "When a test mode helper value is selected from the ring,\nset the tree item's variable to the string value"
        n243 = event-data() -> ("NewVal"=w373:u16)  [unwired: 1 in]
        n244 = property on="Test Ring" class="Ring (strict)"() -> ("Strings []"=w374:string[])  [unwired: 2 in, 2 out]
        n245 = Index Array(array=w374, index=w373) -> (element=w372:string)
        n246 = call <vilib>:"NT Write String.vi"("String"=w372, "Name"=w371) -> ()  [unwired: 9 in, 1 out]
      }
      event "Rec Mode": Value Change {
        # "Update globals for recording mode and path to read log from.\nClear when logging and let NetworkTables set path for vision to\nuse."
        n247 = event-data() -> ("NewVal"=w384:enum32{"Stop", "Record", "Playback"})  [unwired: 1 in]
        n248 = global write "WPI_DashboardLogging Global.vi" "Logging Filename"(path "") -> ()
        n249 = case shown="\"Playback\"" w384 {
          tunnel: w383 -> [_ w386 w394]
          tunnel: [_ _ w393] -> w380
          tunnel: [_ _ w392] -> _
          tunnel: w378 -> [_ _ w390]
          tunnel: cluster{i32, i32} {-250, 170} -> [_ _ w389]
          tunnel: [_ _ T22 {"Image Size"=TRUE, "Image Type"=TRUE, "Pixel Value"=TRUE, "ROI Information"=TRUE, "Zoom Factor"=FALSE} ("Image Information Shown:All Elements")] -> w376
          tunnel: [_ _ TRUE ("Zoom Factor")] -> w375
          frame Default {
          }
          frame "Stop", "Record" {
            # "Place Window too"
            n250 = invoke class="VI" method="FP.Close"(reference=w386) -> (reference out=w385:refnum<vi>)  [unwired: 2 in, 2 out]
            n251 = invoke class="VI" method="Abort VI"(reference=w385) -> ()  [unwired: 2 in, 3 out]
          }
          frame "Playback" {
            n252 = call "Open Playback Panel.vi"("Offset"=w389, "DB VI Ref"=w390, "Playback in"=w394) -> ("Playback out"=w391:refnum<vi>)  [unwired: 8 in]
            n253 = register-events(w391) -> (reference out=w393:refnum<event-registration>, error out=w392:errorcluster)  [unwired: 2 in]
          }
        }
        n254 = global write "WPI_DashboardLogging Global.vi" "Recording"(w384) -> ()
        n255 = property on="Camera Image" class="ImageControl"("Image Information Shown"=w376, "Image Information Visible"=w375) -> ()  [unwired: 2 in, 2 out]
        n256 = call <vilib>:"WPI_DashboardNT Log FieldName Cache.vi"("Operation"=enum16{"Lookup/Add", "Index", "Clear"}."Clear") -> ()  [unwired: 8 in, 3 out]
      }
      event Panel Close {
        w395 = enum32{"Stop", "Record", "Playback"}."Stop" ("Rec Mode")
        # "Playback window has been closed, abort"
        n257 = event-data() -> ()  [unwired: 1 in, 4 out]
        n258 = local write "Rec Mode"(w395) -> ()
        n259 = global write "WPI_DashboardLogging Global.vi" "Recording"(w395) -> ()
      }
      event Panel Close {
        # "Abort playback window and ourself"
        n260 = event-data() -> ()  [unwired: 1 in, 4 out]
        n261 = local read "VISA resource name out"() -> (w399:refnum<visa-resource-name>)
        n262 = VISA Close(VISA resource name=w399) -> (error out=w398:errorcluster)  [unwired: 1 in]
        n263 = call "Shutdown.vi"("error in (no error)"=w398) -> ("error out"=w397:errorcluster)  [unwired: 10 in]
        n264 = invoke class="VI" method="FP.Close"(reference=w403, error in=w397) -> (reference out=w402:refnum<vi>)  [unwired: 1 in, 2 out]
        n265 = invoke class="VI" method="Abort VI"(reference=w402) -> (error out=w401:errorcluster)  [unwired: 2 in, 2 out]
        n266 = invoke class="VI" method="Abort VI"(error in=w401) -> ()  [unwired: 2 in, 3 out]
      }
      event "Vision": Value Change {
        # "Enable/Disable Compression slider.\nHW USB is hard-coded into the camera"
        n267 = event-data() -> ("NewVal"=w409:u16)  [unwired: 1 in]
        n268 = Equal?(x=w409, y=u32 2 ("milliseconds to wait")) -> (x = y?=w407:bool)
        n269 = Select(t=T23."Disabled and Grayed Out" ("Disabled"), s=w407, f=T23."Enabled" ("Disabled")) -> (s? t:f=w404:T23)
        n270 = property on="Compression" class="Slide (strict)"("DisabledEnum"=w404) -> ()  [unwired: 2 in, 2 out]
      }
    }
  }
  n271 = while {
    tunnel: w43 -> [w412]
    i -> [w415]
    stop <- FALSE stop-if-true
    n272 = Wait (ms)(milliseconds to wait=u32 100) -> ()  [unwired: 1 out]
    n273 = case shown="\"Playback\"" "Rec Mode" {
      tunnel: w415 -> [_ _ w430]
      tunnel: [u32 2829099 ("Base Color") u32 11141120 ("Target Color") w419] -> w411
      frame "Stop", Default {
        # "Reset the color, extra updates don't cost much"
      }
      frame "Record" {
      }
      frame "Playback" {
        # "Playback"
        n274 = Quotient & Remainder(x=w430, y=u32 50 ("milliseconds to wait")) -> (x-y*floor(x/y)=w426:u32)  [unwired: 1 out]
        n275 = Divide(x=w426, y=u32 50 ("milliseconds to wait")) -> (x/y=w423:dbl)
        n276 = Multiply(x=6.283185307179586, y=w423) -> (x*y=w428:dbl)
        n277 = Sine(x=w428) -> (sin(x)=w427:dbl)
        n278 = Absolute Value(x=w427) -> (abs(x)=w420:dbl)
        n279 = call "Interpolate RGB Color.vi"("Proportion"=w420, "Target Color"=u32 30976, "Base Color"=u32 2829099) -> ("Result Color"=w419:u32)  [unwired: 8 in]
      }
    }
    n280 = property class="Pane"(reference=w412, "PaneColor"=w411) -> ()  [unwired: 1 in, 2 out]
  }
  n281 = while {
    tunnel: w4 -> [w448]
    tunnel: [w447] -> w3
    tunnel: w2 -> [w431]
    tunnel: w1 -> [_]
    stop <- FALSE stop-if-true
    w443 = FALSE ("element")
    n282 = Build Array("dashButton5", w443, w443, w443, w443, w443) -> (w444:bool[])
    n283 = call-poly <vilib>:"SD Read Value.vi"("Name"="returnBool") -> ("Boolean"=→"Boolean 2":bool)  [unwired: 8 in, 2 out]
    n284 = call "ArduinoSerialReadWrite.vi"("LED"=w444, "VISA resource name"=w448) -> ("error out"=→"error out":errorcluster, "AIs"=w441:dbl[], "Buttons"=w435:bool[], "VISA resource name out"=w447:refnum<visa-resource-name>)  [unwired: 6 in]
    n285 = Index Array(array=w441) -> (element #1=w439:dbl, element #2=w438:dbl)  [unwired: 2 in]
    n286 = Array Subset(array=w435, length=5) -> (w432:bool[])  [unwired: 1 in]
    n287 = call-poly <vilib>:"SD Write Value.vi"("Numeric"=w439, "Name"="dashPot1") -> ()  [unwired: 8 in, 2 out]
    n288 = call-poly <vilib>:"SD Write Value.vi"("Numeric"=w438, "Name"="dashPot2") -> ()  [unwired: 8 in, 2 out]
    n289 = Or Array Elements(Boolean array=w432) -> (logical OR=w433:bool)
    n290 = case shown="True" w433 {
      selector: w433 -> [_ w450]
      tunnel: w432 -> [_ w457]
      tunnel: w431 -> [_ w455]
      frame False {
      }
      frame True {
        n291 = Cluster To Array(cluster=w455) -> (array=w453:dbl[])
        n292 = Search 1D Array(1D array=w457, element=TRUE) -> (index of element=w454:i32)  [unwired: 1 in]
        n293 = Index Array(array=w453, index=w454) -> (element=w452:dbl)
        n294 = call-poly <vilib>:"SD Write Value.vi"("Boolean"=w450, "Name"="PresetButtonPressed") -> ()  [unwired: 8 in, 2 out]
        n295 = call-poly <vilib>:"SD Write Value.vi"("Numeric"=w452, "Name"="PresetValue") -> ()  [unwired: 8 in, 2 out]
      }
    }
  }
  "VISA resource name out" <- w3
  n296 = TCP Create Listener(10:u16 1741 ("timeout ms (25000)")) -> (3:w6:refnum<k5>)  [unwired: 4 in, 2 out]
  n297 = while {
    tunnel: w6 -> [w460]
    stop <- FALSE stop-if-true
    n298 = TCP Wait On Listener(11:w460) -> (4:w459:refnum<k5>)  [unwired: 3 in, 4 out]
    n299 = local write "TCP"(w459) -> ()
  }
  n300 = property on="On/Off" class="Bool (strict)"("Visible"=w11) -> ()  [unwired: 2 in, 2 out]
  n301 = property on="Motor" class="Clust (strict)"("Visible"=w11) -> ()  [unwired: 2 in, 2 out]
  n302 = property on="Progress" class="Clust (strict)"("Visible"=w11) -> ()  [unwired: 2 in, 2 out]
  n303 = property on="Test Ring" class="Ring (strict)"("Visible"=w11) -> ()  [unwired: 2 in, 2 out]
  n304 = property on="Rev/Fwd" class="Clust (strict)"("Visible"=w11) -> ()  [unwired: 2 in, 2 out]
  n305 = property on="Camera Settings" class="Clust (strict)"("Visible"=w11) -> ()  [unwired: 2 in, 2 out]
  n306 = local write "DB Camera Config"(w11) -> ()
  n307 = global write "WPI_DashboardLogging Global.vi" "Recording"(w37) -> ()
  n308 = local write "Rec Mode"(w37) -> ()
